vi "oax_Calculate Runup Phase.vi"(4 "init phase":dbl, 6 "start freq":dbl, 7 "fs":dbl, 8 "post time period":dbl, 9 "middle time period":dbl, 10 "pre time period":dbl, 11 "a":dbl) -> (3 "phase out":dbl[](array[numeric]))   [LabVIEW 2017]
uses:
  <vilib>/Analysis/1siggen.llb/Ramp Pattern by Samples.vi
  <vilib>/Analysis/NI_AALBase.lvlib
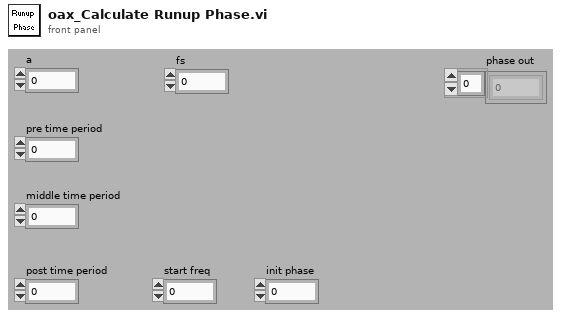
[diagram p1: front panel]
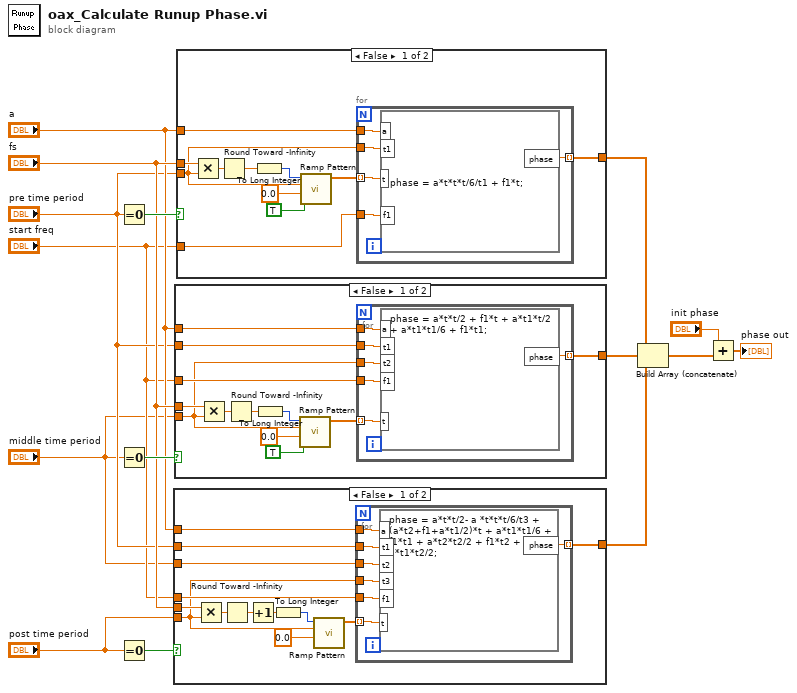
[diagram p0: block diagram]
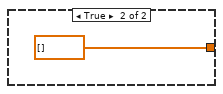
[diagram p2: hidden frame]
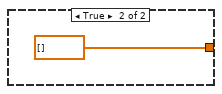
[diagram p3: hidden frame]
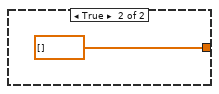
[diagram p4: hidden frame]
diagram:
  n1 = Equal To 0?(x="pre time period") -> (x = 0?=w15:bool)
  n2 = Equal To 0?(x="middle time period") -> (x = 0?=w14:bool)
  n3 = Equal To 0?(x="post time period") -> (x = 0?=w10:bool)
  n4 = case shown="False" w10 {
    tunnel: "fs" -> [w20 _]
    tunnel: "post time period" -> [w16 _]
    tunnel: "a" -> [w25 _]
    tunnel: "middle time period" -> [w23 _]
    tunnel: "pre time period" -> [w24 _]
    tunnel: "start freq" -> [w22 _]
    tunnel: [w21 dbl[] []] -> w5
    frame False {
      n5 = Multiply(x=w20, y=w16) -> (x*y=w26:dbl)
      n6 = Round Toward -Infinity(1:w26) -> (0:w19:dbl)
      n7 = Increment(x=w19) -> (x+1=w18:dbl)
      n8 = To Long Integer(number=w18) -> (32bit integer=w28:i32)
      n9 = call-poly <vilib>:"Ramp Pattern.vi"("start"=0.0, "end"=w16, "samples"=w28) -> ("Ramp Pattern"=w17:dbl[])  [unwired: 7 in, 1 out]
      n10 = for {
        tunnel: w25 -> [w35]
        tunnel: w24 -> [w34]
        tunnel: w23 -> [w33]
        tunnel: w16 -> [w32]
        tunnel: w22 -> [w31]
        tunnel: w17 -> [w30] mode=indexing
        tunnel: [w29] -> w21 mode=indexing
        n11 = formula code="phase = a*t*t/2- a *t*t*t/6/t3 + (a*t2+f1+a*t1/2)*t + a*t1*t1/6 + f1*t1 + a*t2*t2/2 + f1*t2 + a*t1*t2/2;"("a"=w35, "t"=w30, "t1"=w34, "t2"=w33, "t3"=w32, "f1"=w31) -> ("phase"=w29:dbl)
      }
    }
    frame True {
    }
  }
  n12 = case shown="False" w14 {
    tunnel: "fs" -> [w45 _]
    tunnel: "middle time period" -> [w38 _]
    tunnel: "a" -> [w43 _]
    tunnel: "start freq" -> [w41 _]
    tunnel: [w44 dbl[] []] -> w13
    tunnel: "pre time period" -> [w42 _]
    frame False {
      n13 = Multiply(x=w45, y=w38) -> (x*y=w46:dbl)
      n14 = Round Toward -Infinity(1:w46) -> (0:w40:dbl)
      n15 = To Long Integer(number=w40) -> (32bit integer=w48:i32)
      n16 = call-poly <vilib>:"Ramp Pattern.vi"("exclude end?"=TRUE, "start"=0.0, "end"=w38, "samples"=w48) -> ("Ramp Pattern"=w39:dbl[])  [unwired: 6 in, 1 out]
      n17 = for {
        tunnel: w43 -> [w54]
        tunnel: w42 -> [w53]
        tunnel: w38 -> [w52]
        tunnel: w41 -> [w51]
        tunnel: w39 -> [w50] mode=indexing
        tunnel: [w49] -> w44 mode=indexing
        n18 = formula code="phase = a*t*t/2 + f1*t + a*t1*t/2 + a*t1*t1/6 + f1*t1;"("a"=w54, "t"=w50, "t1"=w53, "t2"=w52, "f1"=w51) -> ("phase"=w49:dbl)
      }
    }
    frame True {
    }
  }
  n19 = case shown="False" w15 {
    tunnel: "fs" -> [w63 _]
    tunnel: "pre time period" -> [w57 _]
    tunnel: "a" -> [w61 _]
    tunnel: "start freq" -> [w60 _]
    tunnel: [w62 dbl[] []] -> w12
    frame False {
      n20 = Multiply(x=w63, y=w57) -> (x*y=w64:dbl)
      n21 = Round Toward -Infinity(1:w64) -> (0:w59:dbl)
      n22 = To Long Integer(number=w59) -> (32bit integer=w66:i32)
      n23 = call-poly <vilib>:"Ramp Pattern.vi"("exclude end?"=TRUE, "start"=0.0, "end"=w57, "samples"=w66) -> ("Ramp Pattern"=w58:dbl[])  [unwired: 6 in, 1 out]
      n24 = for {
        tunnel: w61 -> [w71]
        tunnel: w57 -> [w70]
        tunnel: w60 -> [w69]
        tunnel: w58 -> [w68] mode=indexing
        tunnel: [w67] -> w62 mode=indexing
        n25 = formula code="phase = a*t*t*t/6/t1 + f1*t;"("a"=w71, "t"=w68, "t1"=w70, "f1"=w69) -> ("phase"=w67:dbl)
      }
    }
    frame True {
    }
  }
  n26 = Build Array (concatenate)(w12, w13, w5) -> (w11:dbl[])
  n27 = Add(x="init phase", y=w11) -> (x+y=→"phase out":dbl[])
